vi "custom_analog_waveform_generator.vi"() -> ()   [LabVIEW 2025]
uses:
  <vilib>/Utility/file.llb/Read Delimited Spreadsheet (DBL).vi
  <vilib>/measure/maUtilsandCtls.llb/ma_Updatet0 timestamp.vi
  <vilib>/measure/NI_MABase.lvlib
panel:
  out "Points in file":i32
  out "Duration (s)":dbl
  out "Waveform frequency":dbl
  out "Waveform frequency":dbl
  out "Duration (s)":dbl
  out "Points in file":i32
  in  "?":path
  in  "update button":bool
  in  "?":path
  in  "Number of Points":dbl=1000.0 format="%#_13g"
  in  "Sampling rate":dbl=5000.0 format="%#_13g"
  in  "Together ON/OFF":bool
  out "Boolean":bool
  out "Boolean":bool
  in  "Output to DAQ":bool
  out "DAQ Output Voltage":waveform(dbl)[](graph)
  in  "Voltage Amplitude":i32=1
  in  "Voltage Amplitude":i32=1
  in  "stop":bool
  # "Waveform Generator (open-loop)"
  # "X-AXIS"
  # "Y-AXIS"
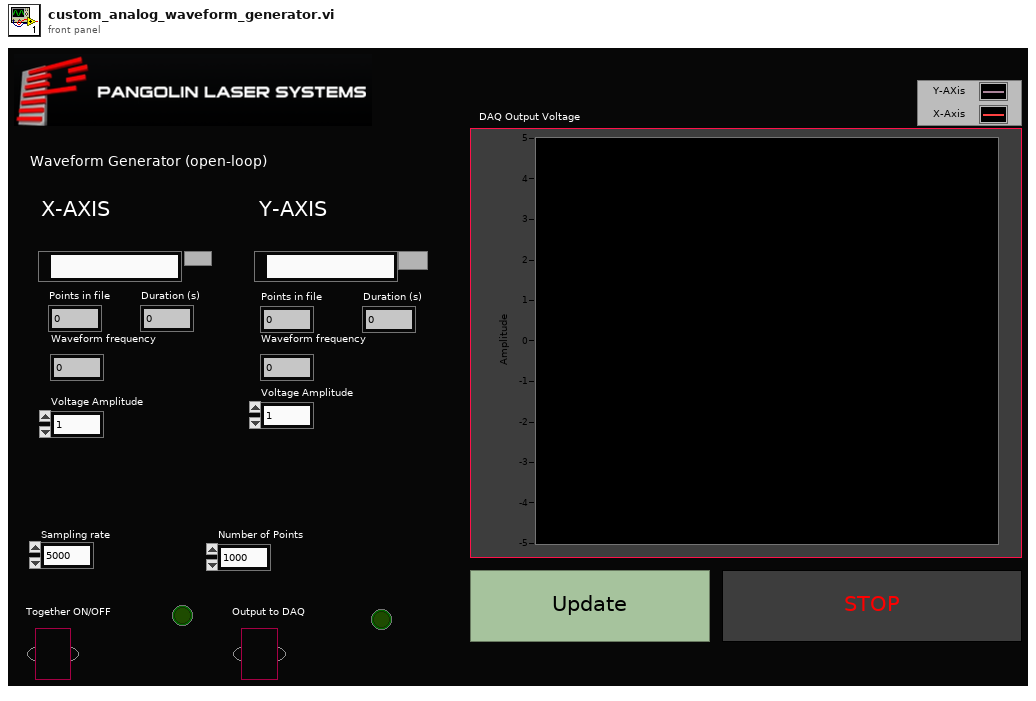
[diagram p1: front panel]
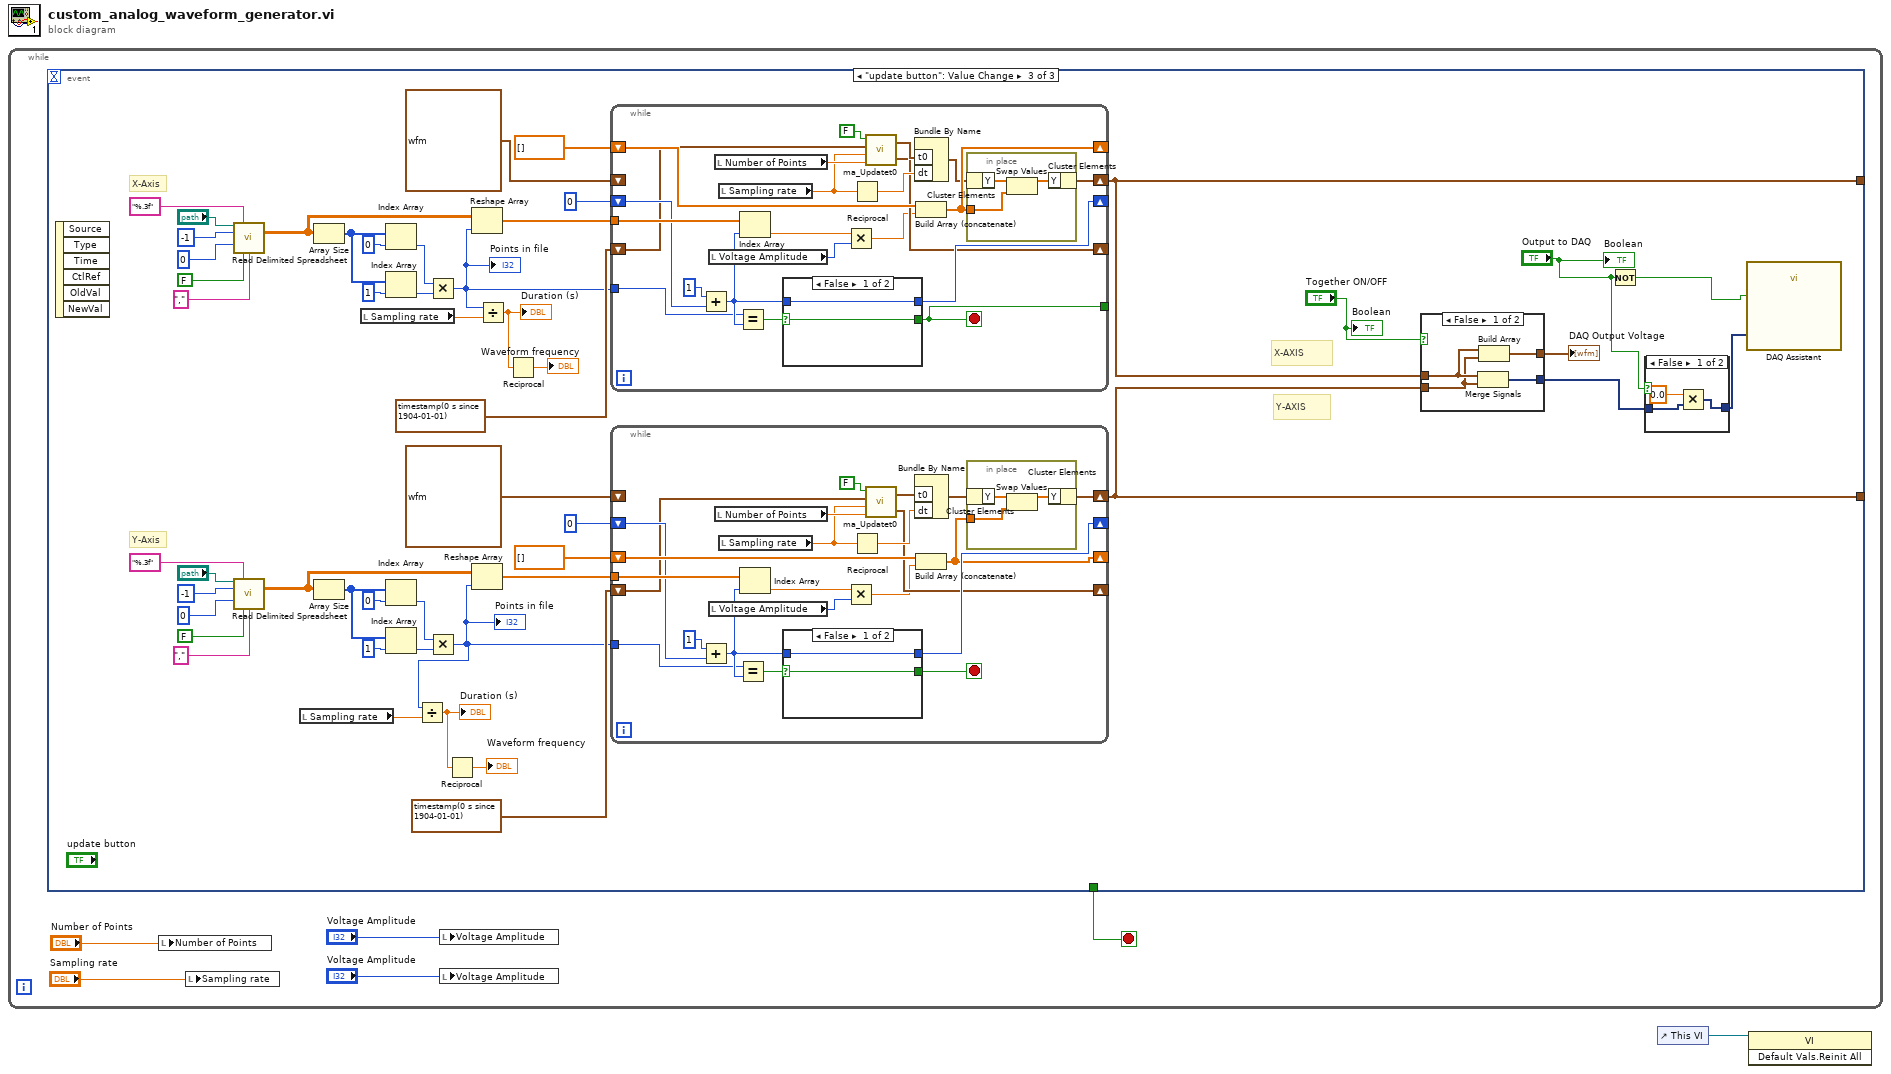
[diagram p0: block diagram]
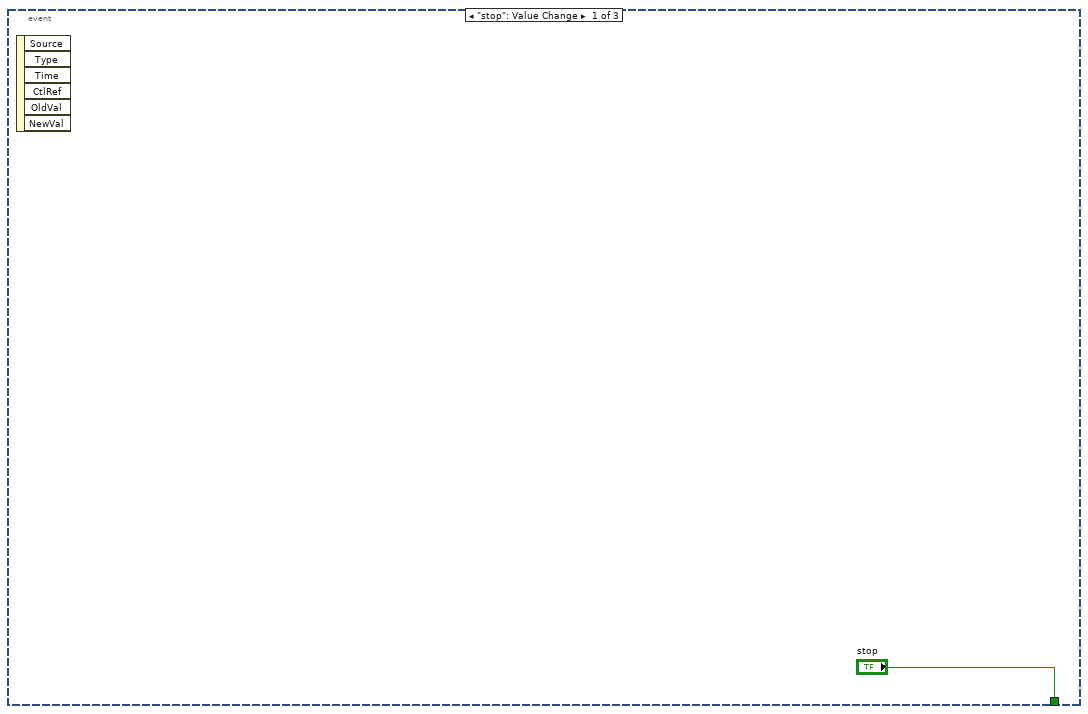
[diagram p2: hidden frame]
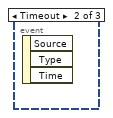
[diagram p3: hidden frame]
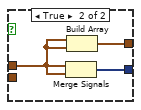
[diagram p5: hidden frame]
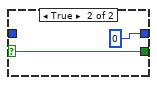
[diagram p6: hidden frame]
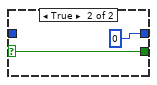
[diagram p7: hidden frame]
diagram:
  n1 = while {
    stop <- w2 stop-if-true
    n2 = event shown="[2] \"update button\": Value Change" {
      selector: _ -> [_ _ _]
      dyn-events: _ -> [_ _ _]
      timeout: _ -> [_ _ _]
      tunnel: [_ _ w40] -> _
      tunnel: [_ _ w22] -> _
      tunnel: ["stop" _ _] -> w2
      event "stop": Value Change {
        n3 = event-data() -> ()  [unwired: 1 in, 6 out]
      }
      event Timeout {
        n4 = event-data() -> ()  [unwired: 1 in, 3 out]
      }
      event "update button": Value Change {
        # "X-AXIS"
        # "Y-AXIS"
        # "Y-Axis"
        # "X-Axis"
        n5 = event-data() -> ()  [unwired: 1 in, 6 out]
        n6 = call-poly <vilib>:"Read Delimited Spreadsheet.vi"("file path (dialog if empty)"="?", "format (%.3f)"="%.3f", "number of rows (all:-1)"=-1, "max characters/row  (no limit:0)"=0, "transpose? (F)"=FALSE, "delimiter (\\t)"="," ("delimiter (\\t)")) -> ("all rows"=w52:dbl[][])  [unwired: 4 in, 5 out]
        n7 = call-poly <vilib>:"Read Delimited Spreadsheet.vi"("file path (dialog if empty)"="?", "format (%.3f)"="%.3f", "number of rows (all:-1)"=-1, "max characters/row  (no limit:0)"=0, "transpose? (F)"=FALSE, "delimiter (\\t)"="," ("delimiter (\\t)")) -> ("all rows"=w34:dbl[][])  [unwired: 4 in, 5 out]
        n8 = local read "Sampling rate"() -> (w13:dbl)
        n9 = Array Size(array=w52) -> (size(s)=w55:i32[])
        n10 = Array Size(array=w34) -> (size(s)=w37:i32[])
        n11 = local read "Sampling rate"() -> (w20:dbl)
        n12 = Index Array(array=w55, index=0) -> (element=w54:i32)
        n13 = Index Array(array=w55, index=1) -> (element=w53:i32)
        n14 = Index Array(array=w37, index=0) -> (element=w36:i32)
        n15 = Index Array(array=w37, index=1) -> (element=w35:i32)
        n16 = Multiply(x=w54, y=w53) -> (x*y=w21:i32)
        "Points in file" <- w21
        n17 = Multiply(x=w36, y=w35) -> (x*y=w12:i32)
        "Points in file" <- w12
        n18 = Divide(x=w12, y=w13) -> (x/y=w14:dbl)
        "Duration (s)" <- w14
        n19 = Reciprocal(x=w14) -> (1/x=→"Waveform frequency":dbl)
        n20 = Reshape Array(w52, w21) -> (w57:dbl[])
        n21 = Reshape Array(w34, w12) -> (w39:dbl[])
        n22 = Divide(x=w21, y=w20) -> (x/y=w19:dbl)
        "Duration (s)" <- w19
        n23 = Reciprocal(x=w19) -> (1/x=→"Waveform frequency":dbl)
        n24 = while {
          shift-right: [w106] -> _
          shift-left: dbl[] [] -> [w116]
          tunnel: w57 -> [w115]
          tunnel: w21 -> [w114]
          shift-right: [w113] -> _
          shift-left: 0 -> [w112]
          shift-right: [w107] -> _
          shift-left: timestamp(0 s since 1904-01-01) ("tf new") -> [w108]
          shift-right: [w104] -> w40
          shift-left: waveform(dbl) {"t0"=timestamp(0 s since 1904-01-01), "dt"=1.0, "Y"=[]} -> [_]
          tunnel: [w98] -> _
          stop <- w98 stop-if-true
          n25 = Add(x=1, y=w112) -> (x+y=w117:i32)
          n26 = local read "Voltage Amplitude"() -> (w99:i32)
          n27 = local read "Number of Points"() -> (w103:dbl)
          n28 = local read "Sampling rate"() -> (w102:dbl)
          n29 = Equal?(x=w114, y=w117) -> (x = y?=w118:bool)
          n30 = Index Array(array=w115, index=w117) -> (element=w101:dbl)
          n31 = case shown="False" w118 {
            selector: w118 -> [w123 w125]
            tunnel: w117 -> [w124 _]
            tunnel: [w124 0] -> w113
            tunnel: [w123 w125] -> w98
            frame False {
            }
            frame True {
            }
          }
          n32 = Multiply(x=w101, y=w99) -> (x*y=w100:dbl)
          n33 = Reciprocal(x=w102) -> (1/x=w110:dbl)
          n34 = call-poly <vilib>:"ma_Updatet0.vi"("samples"=w103, "sampling rate (S/s)"=w102, "tf previous"=w108, "Reset Generation"=FALSE) -> ("tf new"=w107:timestamp, "t0"=w111:timestamp)
          n35 = Bundle By Name("t0"=w111, "dt"=w110) -> (w105:waveform(dbl))  [unwired: 1 in]
          n36 = Build Array (concatenate)(w116, w100) -> (w106:dbl[])
          n37 = in-place {
            in-place-border: w106 -> [w120]
            n38 = in-place-cluster #1(w105) -> ("Y"=w122:dbl[])
            n39 = Swap Values(12:w122, 14:w120) -> (1:w121:dbl[])  [unwired: 1 in, 1 out]
            n40 = in-place-cluster #1("Y"=w121) -> (w104:waveform(dbl))
          }
        }
        n41 = while {
          shift-right: [w77] -> _
          shift-left: dbl[] [] -> [w87]
          tunnel: w39 -> [w86]
          tunnel: w12 -> [w85]
          shift-right: [w84] -> _
          shift-left: 0 -> [w83]
          shift-right: [w78] -> _
          shift-left: timestamp(0 s since 1904-01-01) ("tf new") -> [w79]
          shift-right: [w75] -> w22
          shift-left: waveform(dbl) {"t0"=timestamp(0 s since 1904-01-01), "dt"=1.0, "Y"=[]} -> [_]
          stop <- w69 stop-if-true
          n42 = Add(x=1, y=w83) -> (x+y=w88:i32)
          n43 = local read "Voltage Amplitude"() -> (w70:i32)
          n44 = local read "Number of Points"() -> (w72:dbl)
          n45 = local read "Sampling rate"() -> (w71:dbl)
          n46 = Equal?(x=w85, y=w88) -> (x = y?=w89:bool)
          n47 = Index Array(array=w86, index=w88) -> (element=w74:dbl)
          n48 = case shown="False" w89 {
            selector: w89 -> [w94 w96]
            tunnel: w88 -> [w95 _]
            tunnel: [w95 0] -> w84
            tunnel: [w94 w96] -> w69
            frame False {
            }
            frame True {
            }
          }
          n49 = Multiply(x=w74, y=w70) -> (x*y=w73:dbl)
          n50 = Reciprocal(x=w71) -> (1/x=w81:dbl)
          n51 = call-poly <vilib>:"ma_Updatet0.vi"("samples"=w72, "sampling rate (S/s)"=w71, "tf previous"=w79, "Reset Generation"=FALSE) -> ("tf new"=w78:timestamp, "t0"=w82:timestamp)
          n52 = Bundle By Name("t0"=w82, "dt"=w81) -> (w76:waveform(dbl))  [unwired: 1 in]
          n53 = Build Array (concatenate)(w87, w73) -> (w77:dbl[])
          n54 = in-place {
            in-place-border: w77 -> [w91]
            n55 = in-place-cluster #2(w76) -> ("Y"=w93:dbl[])
            n56 = Swap Values(12:w93, 14:w91) -> (1:w92:dbl[])  [unwired: 1 in, 1 out]
            n57 = in-place-cluster #2("Y"=w92) -> (w75:waveform(dbl))
          }
        }
        n58 = case shown="False" "Together ON/OFF" {
          tunnel: w40 -> [w65 w66]
          tunnel: w22 -> [w64 _]
          tunnel: [w63 w68] -> w11
          tunnel: [w62 w67] -> w16
          frame False {
            n59 = Merge Signals(w65, w64) -> (w63:dynamicdata)
            n60 = Build Array(w65, w64) -> (w62:waveform(dbl)[])
          }
          frame True {
            n61 = Merge Signals(w66, w66) -> (w68:dynamicdata)
            n62 = Build Array(w66, w66) -> (w67:waveform(dbl)[])
          }
        }
        "DAQ Output Voltage" <- w16
        n63 = Not(x="Output to DAQ") -> (.not. x?=w9:bool)
        n64 = case shown="False" "Output to DAQ" {
          tunnel: w11 -> [w60 w61]
          tunnel: [w59 w61] -> w8
          frame False {
            n65 = Multiply(x=0.0, y=w60) -> (x*y=w59:dynamicdata)
          }
          frame True {
          }
        }
        n66 = call "DAQ Assistant"("data"=w8, "stop (F)"=w9) -> ()  [unwired: 15 in, 3 out]
        "Boolean" <- "Together ON/OFF"
        "Boolean" <- "Output to DAQ"
      }
    }
    n67 = local write "Number of Points"("Number of Points") -> ()
    n68 = local write "Sampling rate"("Sampling rate") -> ()
    n69 = local write "Voltage Amplitude"("Voltage Amplitude") -> ()
    n70 = local write "Voltage Amplitude"("Voltage Amplitude") -> ()
  }
  n71 = control-ref of="This VI"() -> (w1:refnum<vi>)
  n72 = invoke class="VI" method="Default Vals.Reinit All"(reference=w1) -> ()  [unwired: 2 in, 3 out]
